vi "DETECTION REPORT for manual.vi"(8 "error in (no error)":errorcluster, 9 "return value 3":cluster{"major":dbl, "minor":dbl, "average":dbl}, 10 "Image File Path":path, 11 "Main Ref":T1) -> (0 "error out":errorcluster)   [LabVIEW 2025]
uses:
  <vilib>/Exaprom PDF/Controls/Font Controls/Font complete cluster.ctl
  <vilib>/Exaprom PDF/Controls/Font Controls/Font size.ctl
  <vilib>/Exaprom PDF/Controls/Font Controls/Font color.ctl
  <vilib>/Exaprom PDF/Controls/Font Controls/Type and encoding.ctl
  <vilib>/Exaprom PDF/Controls/Text Controls/Unicode/Type and run direction.ctl
  <vilib>/Exaprom PDF/Controls/Header, Footer and Watermark Controls/Header or Footer  Text cluster.ctl
  <vilib>/Exaprom PDF/Controls/Table Controls/Cell Alignment 20px.ctl
  <vilib>/Exaprom PDF/Controls/Text Controls/Line spacing.ctl
  <vilib>/Exaprom PDF/Controls/Font Controls/Font complete cluster horizontal.ctl
  <vilib>/Exaprom PDF/Controls/Header, Footer and Watermark Controls/Header or Footer Line cluster.ctl
  <vilib>/Exaprom PDF/Controls/Header, Footer and Watermark Controls/Header Footer Line.ctl
  <vilib>/Exaprom PDF/Controls/Header, Footer and Watermark Controls/Watermark Text Cluster.ctl
  <vilib>/Exaprom PDF/Controls/Header, Footer and Watermark Controls/Watermark Position.ctl
  <vilib>/Exaprom PDF/Controls/Header, Footer and Watermark Controls/Header footer horiz alignment.ctl
  <vilib>/Exaprom PDF/Controls/Image Controls/Image alignment and position.ctl
  <vilib>/Exaprom PDF/Controls/Image Controls/Image aligment.ctl
  <vilib>/Exaprom PDF/Controls/Image Controls/Image border.ctl
  <vilib>/Exaprom PDF/Controls/Table Controls/Table properties.ctl
  <vilib>/Exaprom PDF/Controls/Table Controls/Table position.ctl
  <vilib>/Exaprom PDF/Controls/Header, Footer and Watermark Controls/Header or Footer.ctl
  <vilib>/Exaprom PDF/Controls/Header, Footer and Watermark Controls/Header or Footer  Image cluster.ctl
  <vilib>/Exaprom PDF/Controls/Table Controls/Cell Font, type, Alignment and LS V2.ctl
  <vilib>/Exaprom PDF/Controls/Table Controls/Cell Type, Alignment and LS.ctl
  <vilib>/Exaprom PDF/Controls/Table Controls/Text vertical arrangement.ctl
  <vilib>/Exaprom PDF/VIs/Low level/Header, Footer and Watermark Low level/Append Image HF.vi
  <vilib>/Exaprom PDF/VIs/Low level/Header, Footer and Watermark Low level/Append Text HF.vi
  <vilib>/Exaprom PDF/VIs/Low level/Header, Footer and Watermark Low level/AppendLine seperator.vi
  <vilib>/Exaprom PDF/VIs/Text/Append Phrase.vi
  <vilib>/Exaprom PDF/VIs/Low level/Header, Footer and Watermark Low level/Append Watermark Text.vi
panel:
  in  "Watermark Text 2":T2={"Text "="PALTRO", "Opacity (%)"=5.0, "Position"={"Position"=enum."Center (text section)", "X"=0.0, "Y"=0.0}, "Automatic"=TRUE, "Font"={"Font Name"="", "Size"=-1.0, "Color"=0}, "Alignment"=enum."Center", "Rotate(°)"=0.0}
  in  "Footer Line 2":T7={"H/F Line"=enum."Horizontal line", "Thickness (point)"=0.75, " Colour"=7171459}
  in  "Header Line":T7={"H/F Line"=enum."Horizontal line", "Thickness (point)"=0.75, " Colour"=7171459}
  in  "Footer Text":T9={"Start at page"=1, "Cell Alignment"=4, "Line spacing"=enum."Select", "Text"="Fully automated next-gen fuel and lubricant testers: BOCLE 2.0 , HFRR adv , FBT 3.0", "Font complete"={"Name"="", "Size"=6.0, "Color"=16777224, "Style"={"Bold"=FALSE, "Italic"=FALSE, "Underline"=TRUE, "Strikeout"=FALSE}, "Type"={"Type&direction"=enum."Select", "Embedded"=FALSE, "Encoding"=""}}, "Link"="https://www.paltro.com/products/product-selector/lubricity"}
  in  "Date and Time :":string
  in  "Observations :":string
  in  "Scar Image Path :":path
  in  "Header or footer":T9={"Start at page"=1, "Cell Alignment"=4, "Line spacing"=enum."Select", "Text"="                                            ", "Font complete"={"Name"="", "Size"=-1.0, "Color"=0, "Style"={"Bold"=FALSE, "Italic"=FALSE, "Underline"=FALSE, "Strikeout"=FALSE}, "Type"={"Type&direction"=enum."Select", "Embedded"=FALSE, "Encoding"=""}}, "Link"=""}
  in  "Font":T15={"Name"="", "Size"=18.0, "Color"=0, "Style"={"Bold"=TRUE, "Italic"=FALSE, "Underline"=FALSE, "Strikeout"=FALSE}, "Type"={"Type&direction"=enum."Select", "Embedded"=FALSE, "Encoding"=""}}
  in  "Font 2":T15={"Name"="", "Size"=6.0, "Color"=0, "Style"={"Bold"=FALSE, "Italic"=TRUE, "Underline"=FALSE, "Strikeout"=FALSE}, "Type"={"Type&direction"=enum."Select", "Embedded"=FALSE, "Encoding"=""}}
  in  "File Name :":string(combo)
  out "folder names":string[](array[string])
  out "path out":path
  in  "Automated":bool
  in  "Test Method":string
  in  "Fuel Description":string
  out "Operator :":string
types:
  T1 = cluster{"File Name":string, "Test Method":string, "Operator":string, "Fuel Description":string, "Date and time":string}
  T2 = typedef "Watermark Text Cluster.ctl" = cluster{"Text ":string, "Opacity (%)":sgl, "Position":cluster{"Position":T3, "X":sgl, "Y":sgl}, "Automatic":bool, "Font":cluster{"Font Name":string, "Size":T4, "Color":T5}, "Alignment":T6, "Rotate(°)":sgl}
  T3 = typedef "Watermark Position.ctl" = enum16{"Absolute", "Center (page)", "Center (text section)"}
  T4 = typedef "Font size.ctl" = sgl
  T5 = typedef "Font color.ctl" = u32
  T6 = typedef "Header footer horiz alignment.ctl" = enum16{"Left", "Center", "Right"}
  T7 = typedef "Header or Footer Line cluster.ctl" = cluster{"H/F Line":T8, "Thickness (point)":sgl, " Colour":u32}
  T8 = typedef "Header Footer Line.ctl" = enum16{"No line", "Horizontal line"}
  T9 = typedef "Header or Footer  Text cluster.ctl" = cluster{"Start at page":i32, "Cell Alignment":T10, "Line spacing":T11, "Text":string, "Font complete":T12, "Link":string}
  T10 = typedef "Cell Alignment 20px.ctl" = u16
  T11 = typedef "Line spacing.ctl" = enum16{"Select", "1.0", "1.5", "2.0"}
  T12 = typedef "Font complete cluster horizontal.ctl" = cluster{"Name":string, "Size":T4, "Color":T5, "Style":cluster{"Bold":bool, "Italic":bool, "Underline":bool, "Strikeout":bool}, "Type":T13}
  T13 = typedef "Type and encoding.ctl" = cluster{"Type&direction":T14, "Embedded":bool, "Encoding":string}
  T14 = typedef "Type and run direction.ctl" = enum16{"Select", "ASCII", "UTF-16", "UTF-16 (default)", "UTF-16 (LTR)", "UTF-16 (RTL)"}
  T15 = typedef "Font complete cluster.ctl" = cluster{"Name":string, "Size":T4, "Color":T5, "Style":cluster{"Bold":bool, "Italic":bool, "Underline":bool, "Strikeout":bool}, "Type":T13}
  T16 = typedef "Cell Font, type, Alignment and LS V2.ctl" = cluster{"Cell Type, Alignment and LS":T17, "Font":T15}
  T17 = typedef "Cell Type, Alignment and LS.ctl" = cluster{"Cell Alignment":T10, "Text rotation":T18, "Line spacing":T11}
  T18 = typedef "Text vertical arrangement.ctl" = enum16{"None", "Clockwise", "Counterclockwise"}
  T19 = typedef "Header or Footer  Image cluster.ctl" = cluster{"Start at page":i32, "Cell Alignment":T10, "Path":path, "Image (%)":sgl, "Link":string}
  T20 = typedef "Image alignment and position.ctl" = cluster{"Alignment":T21, "X ":sgl, "Y":sgl, "Indentation":sgl}
  T21 = typedef "Image aligment.ctl" = enum16{"Absolute (X,Y)", "Left", "Center", "Right", "Left (textwrap)", "Right (textwrap)"}
  T22 = typedef "Image border.ctl" = cluster{"Show?":bool, "Thickness (point)":sgl, "Color":u32}
  T23 = typedef "Table properties.ctl" = cluster{"Table position":T24, "SpacingBefore (points)":sgl, "SpacingAfter (points)":sgl}
  T24 = typedef "Table position.ctl" = i32
  T25 = typedef "Header or Footer.ctl" = enum16{"Header", "Footer"}
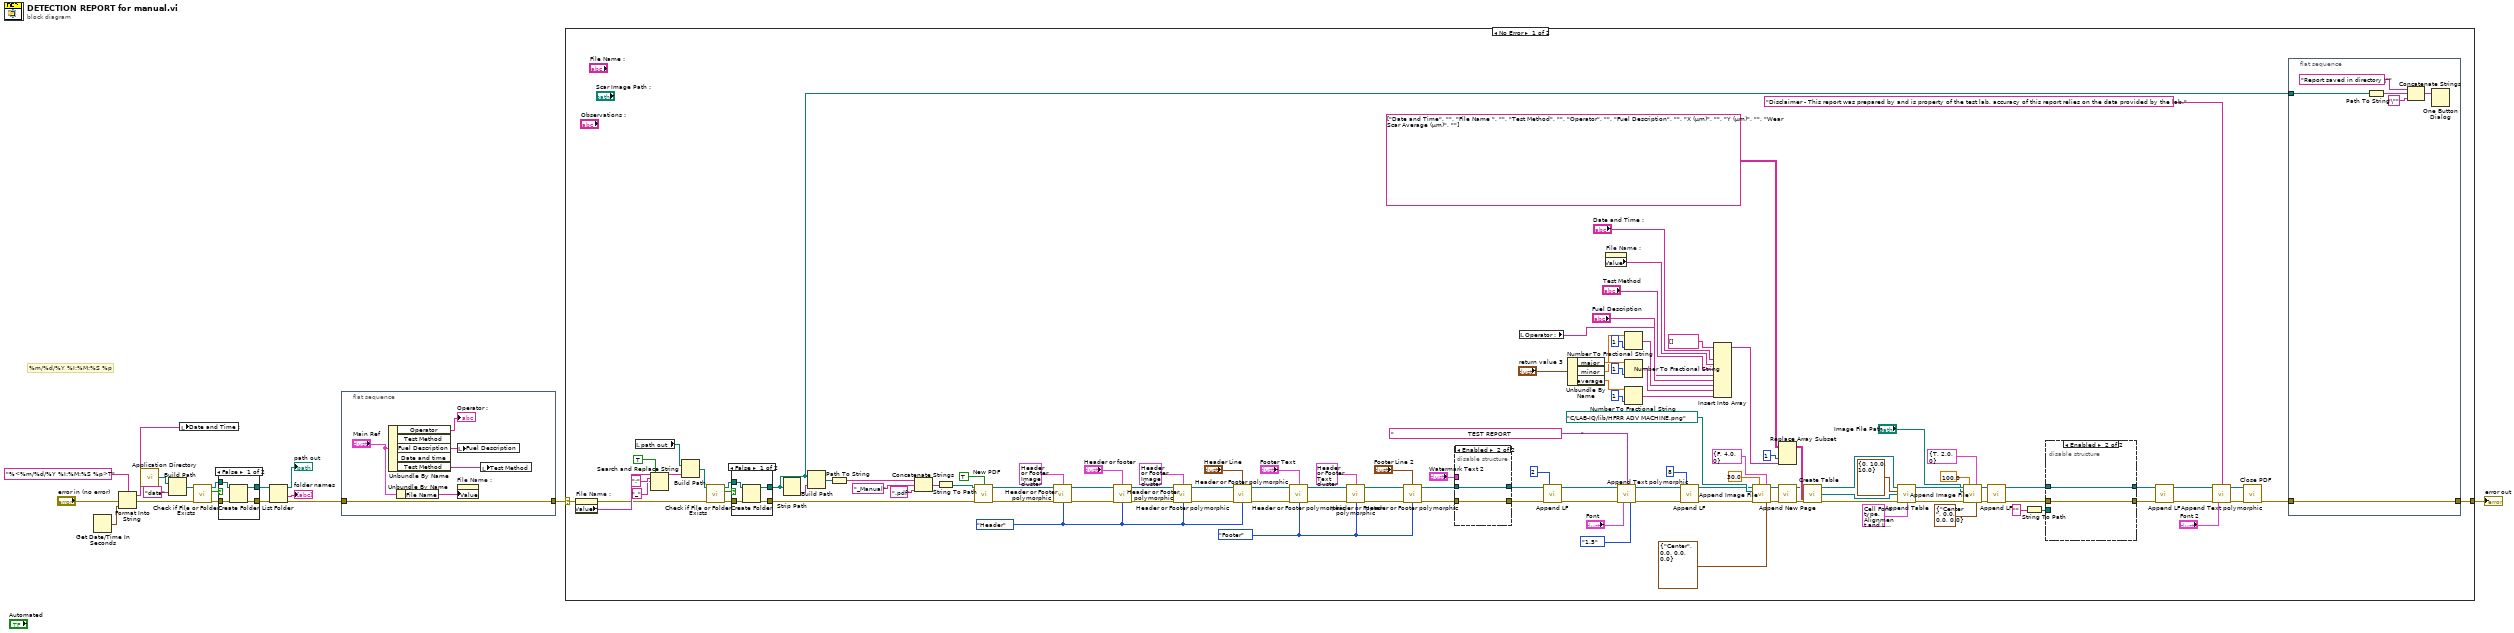
[diagram p0: block diagram]
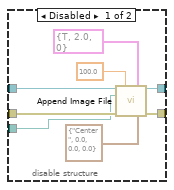
[diagram p2: hidden frame]
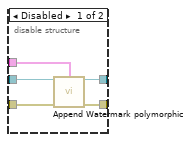
[diagram p3: hidden frame]
diagram:
  # "%m/%d/%Y %I:%M:%S %p"
  n1 = Get Date/Time In Seconds() -> (seconds since 1Jan1904=w7:timestamp)
  n2 = Format Into String(format string="%<%m/%d/%Y %I:%M:%S %p>T", error in="error in (no error)", w7) -> (resulting string=w1:string, error out=w5:errorcluster)  [unwired: 1 in]
  n3 = call <vilib>:"Application Directory.vi"() -> ("Application Directory"=w9:path)
  n4 = Build Path(base path=w9, name or relative path="data") -> (appended path=w8:path)
  n5 = local write "Date and Time :"(w1) -> ()
  n6 = call <vilib>:"Check if File or Folder Exists.vi"("error in (no error)"=w5, "path"=w8) -> ("error out"=w13:errorcluster, "file or folder exists?"=w15:bool, "dup path"=w14:path)  [unwired: 7 in]
  n7 = case shown="False" w15 {
    tunnel: w14 -> [w22 w23]
    tunnel: w13 -> [w21 w24]
    tunnel: [w20 w24] -> w18
    tunnel: [w19 w23] -> w16
    frame False {
      n8 = Create Folder(path (use dialog)=w22, error in=w21) -> (created path=w19:path, error out=w20:errorcluster)  [unwired: 1 in, 1 out]
    }
    frame True {
    }
  }
  n9 = List Folder(path=w16, error in=w18) -> (path out=→"path out":path, folder names=→"folder names":string[], error out=w3:errorcluster)  [unwired: 2 in, 1 out]
  n10 = flat-sequence {
    tunnel: w3 -> [w26]
    tunnel: [w26] -> w2
    frame #0 {
      n11 = Unbundle By Name("Main Ref") -> ("Operator"=→"Operator :":string, "Fuel Description"=w27:string, "Test Method"=w25:string)  [unwired: 2 out]
      n12 = Unbundle By Name("Main Ref") -> ("File Name"=w30:string)
      n13 = local write "Fuel Description"(w27) -> ()
      n14 = property on="File Name :" class="CmbBox"("Value"=w30) -> ()  [unwired: 2 in, 2 out]
      n15 = local write "Test Method"(w25) -> ()
    }
  }
  n16 = case shown="No Error" w2 {
    selector: w2 -> [w55 _]
    tunnel: [w51 _] -> w11
    frame No Error {
      w70 = Header_or_Footer."Header" ("Position")
      w100 = Header_or_Footer."Footer" ("Position")
      n17 = property on="File Name :" class="CmbBox"(error in=w55) -> (error out=w59:errorcluster, "Value"=w60:string)  [unwired: 1 in, 1 out]
      n18 = local read "path out"() -> (w61:path)
      n19 = Search and Replace String(replace all?=TRUE ("replace all? (F)"), input string=w60, search string=":", replace string="_" ("replace string (\"\")")) -> (result string=w90:string)  [unwired: 4 in, 3 out]
      n20 = Build Path(base path=w61, name or relative path=w90) -> (appended path=w117:path)
      n21 = call <vilib>:"Check if File or Folder Exists.vi"("error in (no error)"=w59, "path"=w117) -> ("error out"=w114:errorcluster, "file or folder exists?"=w116:bool, "dup path"=w115:path)  [unwired: 7 in]
      n22 = case shown="False" w116 {
        tunnel: w115 -> [w173 w174]
        tunnel: w114 -> [w172 w175]
        tunnel: [w171 w175] -> w113
        tunnel: [w170 w174] -> w62
        frame False {
          n23 = Create Folder(path (use dialog)=w173, error in=w172) -> (created path=w170:path, error out=w171:errorcluster)  [unwired: 1 in, 1 out]
        }
        frame True {
        }
      }
      n24 = Strip Path(path=w62) -> (name=w119:string)  [unwired: 1 out]
      n25 = Build Path(base path=w62, name or relative path=w119) -> (appended path=w118:path)
      n26 = Path To String(path=w118) -> (string=w50:string)
      n27 = Concatenate Strings(w50, "_Manual" ("string"), ".pdf" ("string")) -> (w120:string)
      n28 = String To Path(string=w120) -> (path=w112:path)
      n29 = call <vilib>:"New PDF.vi"("PDF Path"=w112, "Overwrite?"=TRUE, "error in (no error)"=w113) -> ("PDF Report"=w134:refnum<class "PDF Report Class.lvclass">, "error out"=w135:errorcluster)  [unwired: 11 in]
      n30 = call-poly <vilib>:"Header or Footer polymorphic.vi"("PDF Report IN"=w134, "Header or footer"=T19 {"Start at page"=1, "Cell Alignment"=4, "Path"=path "C:/LAB-IQ/lib/paltro logo.png", "Image (%)"=100.0, "Link"="https://www.paltro.com/"} ("HEADER Image"), "error in (no error)"=w135, "Position"=w70) -> ("PDF Report OUT"=w88:refnum<class "PDF Report Class.lvclass">, "error out"=w89:errorcluster)  [unwired: 10 out]
      n31 = call-poly <vilib>:"Header or Footer polymorphic.vi"("PDF Report IN"=w88, "Header or footer"="Header or footer", "error in (no error)"=w89, "Position"=w70) -> ("PDF Report OUT"=w86:refnum<class "PDF Report Class.lvclass">, "error out"=w87:errorcluster)  [unwired: 10 out]
      n32 = call-poly <vilib>:"Header or Footer polymorphic.vi"("PDF Report IN"=w86, "Header or footer"=T19 {"Start at page"=1, "Cell Alignment"=6, "Path"=path "C:/LAB-IQ/lib/HFRR_adv.png", "Image (%)"=30.0, "Link"="https://www.paltro.com/products/test-and-measurement/bocle--automated-ball-on-cylinder-lubricity-evaluator"} ("HEADER Image  2"), "error in (no error)"=w87, "Position"=w70) -> ("PDF Report OUT"=w106:refnum<class "PDF Report Class.lvclass">, "error out"=w107:errorcluster)  [unwired: 10 out]
      n33 = call-poly <vilib>:"Header or Footer polymorphic.vi"("PDF Report IN"=w106, "H/F Line"="Header Line", "error in (no error)"=w107, "Position"=w70) -> ("PDF Report OUT"=w138:refnum<class "PDF Report Class.lvclass">, "error out"=w137:errorcluster)  [unwired: 1 in, 9 out]
      n34 = call-poly <vilib>:"Header or Footer polymorphic.vi"("PDF Report IN"=w138, "Header or footer"="Footer Text", "error in (no error)"=w137, "Position"=w100) -> ("PDF Report OUT"=w140:refnum<class "PDF Report Class.lvclass">, "error out"=w139:errorcluster)  [unwired: 10 out]
      n35 = call-poly <vilib>:"Header or Footer polymorphic.vi"("PDF Report IN"=w140, "Header or footer"=T9 {"Start at page"=1, "Cell Alignment"=6, "Line spacing"=enum."Select", "Text"="www.paltro.com", "Font complete"={"Name"="", "Size"=6.0, "Color"=16777224, "Style"={"Bold"=FALSE, "Italic"=FALSE, "Underline"=TRUE, "Strikeout"=FALSE}, "Type"={"Type&direction"=enum."Select", "Embedded"=FALSE, "Encoding"=""}}, "Link"="https://www.paltro.com/"} ("Footer Text 2"), "error in (no error)"=w139, "Position"=w100) -> ("PDF Report OUT"=w133:refnum<class "PDF Report Class.lvclass">, "error out"=w132:errorcluster)  [unwired: 10 out]
      n36 = call-poly <vilib>:"Header or Footer polymorphic.vi"("PDF Report IN"=w133, "H/F Line"="Footer Line 2", "error in (no error)"=w132, "Position"=w100) -> ("PDF Report OUT"=w126:refnum<class "PDF Report Class.lvclass">, "error out"=w127:errorcluster)  [unwired: 1 in, 9 out]
      n37 = disable-structure shown="Enabled" {
        disable-tunnel: "Watermark Text 2" -> [w167 _]
        disable-tunnel: w127 -> [w166 w169]
        disable-tunnel: w126 -> [w165 w168]
        disable-tunnel: [w164 w169] -> w82
        disable-tunnel: [w163 w168] -> w81
        frame Disabled {
          n38 = call-poly <vilib>:"Append Watermark polymorphic.vi"("PDF Report IN"=w165, "Watermark Text"=w167, "error in (no error)"=w166) -> ("PDF Report OUT"=w163:refnum<class "PDF Report Class.lvclass">, "error out"=w164:errorcluster)  [unwired: 1 in, 10 out]
        }
        frame Enabled {
        }
      }
      n39 = local read "Operator :"() -> (w31:string)
      n40 = call <vilib>:"Append LF.vi"("PDF Report IN"=w81, "Number of LF (default 1)"=u8 2, "error in (no error)"=w82) -> ("PDF Report duplicate"=w79:refnum<class "PDF Report Class.lvclass">, "error out"=w80:errorcluster)  [unwired: 11 in]
      n41 = Unbundle By Name("return value 3") -> ("major"=w34:dbl, "minor"=w33:dbl, "average"=w32:dbl)
      n42 = property on="File Name :" class="CmbBox"() -> ("Value"=w58:string)  [unwired: 2 in, 2 out]
      n43 = call-poly <vilib>:"Append Text polymorphic.vi"("PDF Report IN"=w79, "Text"="                                     TEST REPORT                                   ", "error in (no error)"=w80, "Font"="Font", "Line spacing"=Line_spacing."1.5") -> ("PDF Report OUT"=w66:refnum<class "PDF Report Class.lvclass">, "error out"=w67:errorcluster)  [unwired: 9 in]
      n44 = Number To Fractional String(number=w33, precision (6)=i16 1) -> (F-format string=w38:string)  [unwired: 2 in]
      n45 = Number To Fractional String(number=w34, precision (6)=i16 1) -> (F-format string=w39:string)  [unwired: 2 in]
      n46 = Number To Fractional String(number=w32, precision (6)=i16 1) -> (F-format string=w40:string)  [unwired: 2 in]
      n47 = call <vilib>:"Append LF.vi"("PDF Report IN"=w66, "Number of LF (default 1)"=u8 8, "error in (no error)"=w67) -> ("PDF Report duplicate"=w69:refnum<class "PDF Report Class.lvclass">, "error out"=w68:errorcluster)  [unwired: 11 in]
      n48 = Insert Into Array(array=string[] [], new element #1="Date and Time :", new element #2=w58, new element #3="Test Method", new element #4=w31, new element #5="Fuel Description", new element #6=w38, new element #7=w39, new element #8=w40) -> (w142:string[])  [unwired: 1 in]
      n49 = call <vilib>:"Append Image File.vi"("PDF Report IN"=w69, "Scale (%)"=sgl 30.0, "Border"=T22 {"Show?"=FALSE, "Thickness (point)"=4.0, "Color"=0}, "Image path"=path "C:/LAB-IQ/lib/HFRR ADV MACHINE.png", "error in (no error)"=w68, "Position and indentation"=T20 {"Alignment"=enum."Center", "X "=0.0, "Y"=0.0, "Indentation"=0.0}) -> ("PDF Report OUT"=w110:refnum<class "PDF Report Class.lvclass">, "error out"=w111:errorcluster)  [unwired: 6 in, 2 out]
      n50 = Replace Array Subset(array=string[][] [["Date and Time", ""], ["File Name ", ""], ["Test Method", ""], ["Operator", ""], ["Fuel Description", ""], ["X (µm)", ""], ["Y (µm)", ""], ["Wear Scar Average (µm)", ""]] ("Text Data 2D [ ]"), new element=w142, index (col)=1 ("disabled index (col)")) -> (w143:string[][])  [unwired: 1 in]
      n51 = call <vilib>:"Append New Page.vi"("PDF Report"=w110, "error in (no error)"=w111) -> ("PDF Report duplicate"=w108:refnum<class "PDF Report Class.lvclass">, "error OUT"=w109:errorcluster)  [unwired: 12 in]
      n52 = call <vilib>:"Create Table.vi"("PDF Report IN"=w108, "Text Data 2D [ ]"=w143, "error in (no error)"=w109) -> ("PDF Report duplicate"=w123:refnum<class "PDF Report Class.lvclass">, "PDF Table"=w125:refnum<class "Pdfp Table Class.lvclass">, "error out"=w121:errorcluster)  [unwired: 10 in]
      n53 = call <vilib>:"Append Table.vi"("PDF Report IN"=w123, "Table properties"=T23 {"Table position"=0, "SpacingBefore (points)"=10.0, "SpacingAfter (points)"=10.0} ("Table properties  - Tables 2 to 4"), "PDF Table"=w125, "error in (no error)"=w121, "Datas format"=T16 {"Cell Type, Alignment and LS"={"Cell Alignment"=4, "Text rotation"=enum."None", "Line spacing"=enum."Select"}, "Font"={"Name"="", "Size"=-1.0, "Color"=0, "Style"={"Bold"=FALSE, "Italic"=FALSE, "Underline"=FALSE, "Strikeout"=FALSE}, "Type"={"Type&direction"=enum."Select", "Embedded"=FALSE, "Encoding"=""}}}) -> ("PDF Report OUT"=w124:refnum<class "PDF Report Class.lvclass">, "error out"=w122:errorcluster)  [unwired: 7 in, 2 out]
      n54 = call <vilib>:"Append Image File.vi"("PDF Report IN"=w124, "Scale (%)"=sgl 100.0, "Border"=T22 {"Show?"=TRUE, "Thickness (point)"=2.0, "Color"=0}, "Image path"="Image File Path", "error in (no error)"=w122, "Position and indentation"=T20 {"Alignment"=enum."Center", "X "=0.0, "Y"=0.0, "Indentation"=0.0}) -> ("PDF Report OUT"=w72:refnum<class "PDF Report Class.lvclass">, "error out"=w73:errorcluster)  [unwired: 6 in, 2 out]
      n55 = call <vilib>:"Append LF.vi"("PDF Report IN"=w72, "error in (no error)"=w73) -> ("PDF Report duplicate"=w44:refnum<class "PDF Report Class.lvclass">, "error out"=w45:errorcluster)  [unwired: 12 in]
      n56 = String To Path(string="") -> (path=w41:path)
      n57 = disable-structure shown="Enabled" {
        disable-tunnel: [w154 w156] -> w47
        disable-tunnel: [w153 w155] -> w46
        disable-tunnel: w45 -> [w150 w155]
        disable-tunnel: w44 -> [w149 w156]
        disable-tunnel: w41 -> [w147 _]
        frame Disabled {
          n58 = call <vilib>:"Append Image File.vi"("PDF Report IN"=w149, "Scale (%)"=sgl 100.0, "Border"=T22 {"Show?"=TRUE, "Thickness (point)"=2.0, "Color"=0}, "Image path"=w147, "error in (no error)"=w150, "Position and indentation"=T20 {"Alignment"=enum."Center", "X "=0.0, "Y"=0.0, "Indentation"=0.0}) -> ("PDF Report OUT"=w154:refnum<class "PDF Report Class.lvclass">, "error out"=w153:errorcluster)  [unwired: 6 in, 2 out]
        }
        frame Enabled {
        }
      }
      n59 = call <vilib>:"Append LF.vi"("PDF Report IN"=w47, "error in (no error)"=w46) -> ("PDF Report duplicate"=w42:refnum<class "PDF Report Class.lvclass">, "error out"=w43:errorcluster)  [unwired: 12 in]
      n60 = call-poly <vilib>:"Append Text polymorphic.vi"("PDF Report IN"=w42, "Text"="Disclaimer - This report was prepared by and is property of the test lab, accuracy of this report relies on the data provided by the lab.", "error in (no error)"=w43, "Font"="Font 2") -> ("PDF Report OUT"=w75:refnum<class "PDF Report Class.lvclass">, "error out"=w76:errorcluster)  [unwired: 10 in]
      n61 = call <vilib>:"Close PDF.vi"("PDF Report"=w75, "error in (no error)"=w76) -> ("error out"=w63:errorcluster)  [unwired: 12 in, 1 out]
      n62 = flat-sequence {
        tunnel: w63 -> [w162]
        tunnel: [w162] -> w51
        tunnel: w62 -> [w161]
        frame #0 {
          n63 = Path To String(path=w161) -> (string=w160:string)
          n64 = Concatenate Strings("Report saved in directory \"", w160, "\"" ("string")) -> (w157:string)
          n65 = One Button Dialog(message=w157) -> ()  [unwired: 1 in, 1 out]
        }
      }
    }
    frame Error {
      # "WHEN USER PRESSED CLOSE BUTTON"
    }
  }
  "error out" <- w11
